vi "Open Pneumatics.vi"(9 "PCM CAN ID":u8) -> ()   [LabVIEW 2018]
uses:
  <vilib>/Rock Robotics/WPI/Solenoid/WPI_SolenoidChannel.ctl
  <vilib>/Rock Robotics/WPI/Solenoid/WPI_SolenoidValue.ctl
  <vilib>/Rock Robotics/WPI/Solenoid/WPI_SolenoidOpenDouble.vi
  <vilib>/Rock Robotics/WPI/Utilities/WPI_GetSetVariantRefNum.vi
  <vilib>/Rock Robotics/WPI/Solenoid/WPI_SolenoidSetEnum.vi
  <vilib>/Rock Robotics/WPI/Solenoid/WPI_SolenoidOpenSingle.vi
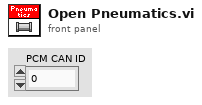
[diagram p1: front panel]
types:
  T1 = typedef "WPI_SolenoidValue.ctl" = enum16{"Off", "On", "Forward", "Reverse"}
  T2 = typedef "WPI_SolenoidChannel.ctl" = enum8{"Solenoid 0", "Solenoid 1", "Solenoid 2", "Solenoid 3", "Solenoid 4", "Solenoid 5", "Solenoid 6", "Solenoid 7", "Invalid"}
  T3 = typedef "WPI_SolenoidDevRef.ctl" = cluster{"DevStatus":errorcluster, "Pneumatics Control Module":u8, "Forward Solenoid Channel":T2, "Reverse Solenoid Channel":T2}
  T4 = typedef "WPI_CompressorDevRef.ctl" = cluster{"DevStatus":errorcluster, "Pneumatics Control Module":u8}
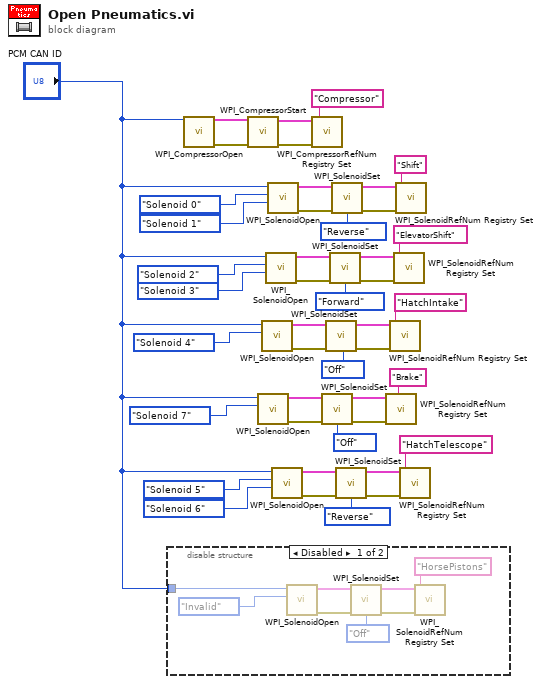
[diagram p0: block diagram]
diagram:
  n1 = disable-structure shown="Disabled" {
    disable-tunnel: "PCM CAN ID" -> [w45 _]
    frame Disabled {
      n2 = call-poly <vilib>:"WPI_SolenoidOpen.vi"("Solenoid Channel"=WPI_SolenoidChannel."Invalid", "Pneumatics Control Module (0)"=w45) -> ("error out"=w48:errorcluster, "SolenoidDevRef"=w49:T3)  [unwired: 8 in]
      n3 = call-poly <vilib>:"WPI_SolenoidSet.vi"("error in (no error)"=w48, "Value"=WPI_SolenoidValue."Off", "SolenoidDevRef"=w49) -> ("error out"=w47:errorcluster, "SolenoidDevRef"=w50:T3)  [unwired: 7 in]
      n4 = call <vilib>:"WPI_SolenoidRefNum Registry Set.vi"("error in (no error)"=w47, "refnum name"="HorsePistons", "SolenoidDevRef"=w50) -> ()  [unwired: 7 in, 2 out]
    }
    frame Enabled {
    }
  }
  n5 = call <vilib>:"WPI_CompressorOpen.vi"("Pneumatics Control Module (0)"="PCM CAN ID") -> ("CompressorDevRef"=w42:T4, "error out"=w41:errorcluster)  [unwired: 13 in]
  n6 = call <vilib>:"WPI_CompressorStart.vi"("error in (no error)"=w41, "CompressorDevRef"=w42) -> ("error out"=w44:errorcluster, "CompressorDevRef"=w43:T4)  [unwired: 8 in]
  n7 = call-poly <vilib>:"WPI_SolenoidOpen.vi"("Solenoid Channel"=WPI_SolenoidChannel."Solenoid 7", "Pneumatics Control Module (0)"="PCM CAN ID") -> ("error out"=w20:errorcluster, "SolenoidDevRef"=w22:T3)  [unwired: 8 in]
  n8 = call-poly <vilib>:"WPI_SolenoidOpen.vi"("Solenoid Channel"=WPI_SolenoidChannel."Solenoid 4", "Pneumatics Control Module (0)"="PCM CAN ID") -> ("error out"=w13:errorcluster, "SolenoidDevRef"=w10:T3)  [unwired: 8 in]
  n9 = call-poly <vilib>:"WPI_SolenoidOpen.vi"("Reverse Solenoid Channel"=WPI_SolenoidChannel."Solenoid 3", "Forward Solenoid Channel"=WPI_SolenoidChannel."Solenoid 2" ("Solenoid Channel"), "Pneumatics Control Module (0)"="PCM CAN ID") -> ("error out"=w27:errorcluster, "SolenoidDevRef"=w31:T3)  [unwired: 7 in]
  n10 = call-poly <vilib>:"WPI_SolenoidOpen.vi"("Reverse Solenoid Channel"=WPI_SolenoidChannel."Solenoid 1", "Forward Solenoid Channel"=WPI_SolenoidChannel."Solenoid 0", "Pneumatics Control Module (0)"="PCM CAN ID") -> ("error out"=w29:errorcluster, "SolenoidDevRef"=w33:T3)  [unwired: 7 in]
  n11 = call-poly <vilib>:"WPI_SolenoidOpen.vi"("Reverse Solenoid Channel"=WPI_SolenoidChannel."Solenoid 6", "Forward Solenoid Channel"=WPI_SolenoidChannel."Solenoid 5", "Pneumatics Control Module (0)"="PCM CAN ID") -> ("error out"=w11:errorcluster, "SolenoidDevRef"=w7:T3)  [unwired: 7 in]
  n12 = call <vilib>:"WPI_CompressorRefNum Registry Set.vi"("error in (no error)"=w44, "refnum name"="Compressor", "CompressorDevRef"=w43) -> ()  [unwired: 7 in, 2 out]
  n13 = call-poly <vilib>:"WPI_SolenoidSet.vi"("error in (no error)"=w20, "Value"=WPI_SolenoidValue."Off", "SolenoidDevRef"=w22) -> ("error out"=w19:errorcluster, "SolenoidDevRef"=w21:T3)  [unwired: 7 in]
  n14 = call-poly <vilib>:"WPI_SolenoidSet.vi"("error in (no error)"=w13, "Value"=WPI_SolenoidValue."Off", "SolenoidDevRef"=w10) -> ("error out"=w14:errorcluster, "SolenoidDevRef"=w9:T3)  [unwired: 7 in]
  n15 = call-poly <vilib>:"WPI_SolenoidSet.vi"("error in (no error)"=w27, "Value"=WPI_SolenoidValue."Forward", "SolenoidDevRef"=w31) -> ("error out"=w26:errorcluster, "SolenoidDevRef"=w30:T3)  [unwired: 7 in]
  n16 = call-poly <vilib>:"WPI_SolenoidSet.vi"("error in (no error)"=w29, "Value"=WPI_SolenoidValue."Reverse", "SolenoidDevRef"=w33) -> ("error out"=w28:errorcluster, "SolenoidDevRef"=w32:T3)  [unwired: 7 in]
  n17 = call-poly <vilib>:"WPI_SolenoidSet.vi"("error in (no error)"=w11, "Value"=WPI_SolenoidValue."Reverse", "SolenoidDevRef"=w7) -> ("error out"=w12:errorcluster, "SolenoidDevRef"=w8:T3)  [unwired: 7 in]
  n18 = call <vilib>:"WPI_SolenoidRefNum Registry Set.vi"("error in (no error)"=w19, "refnum name"="Brake", "SolenoidDevRef"=w21) -> ()  [unwired: 7 in, 2 out]
  n19 = call <vilib>:"WPI_SolenoidRefNum Registry Set.vi"("error in (no error)"=w14, "refnum name"="HatchIntake", "SolenoidDevRef"=w9) -> ()  [unwired: 7 in, 2 out]
  n20 = call <vilib>:"WPI_SolenoidRefNum Registry Set.vi"("error in (no error)"=w26, "refnum name"="ElevatorShift", "SolenoidDevRef"=w30) -> ()  [unwired: 7 in, 2 out]
  n21 = call <vilib>:"WPI_SolenoidRefNum Registry Set.vi"("error in (no error)"=w28, "refnum name"="Shift", "SolenoidDevRef"=w32) -> ()  [unwired: 7 in, 2 out]
  n22 = call <vilib>:"WPI_SolenoidRefNum Registry Set.vi"("error in (no error)"=w12, "refnum name"="HatchTelescope", "SolenoidDevRef"=w8) -> ()  [unwired: 7 in, 2 out]
